vi "wait.vi"(8 "error_in":errorcluster, 11 "milliseconds_to_wait":u32) -> (0 "error_out":errorcluster)   [LabVIEW 2019]
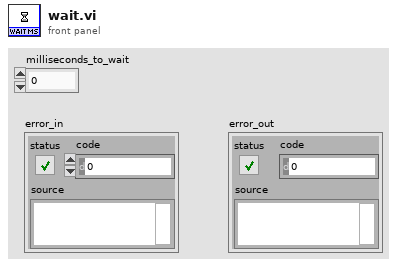
[diagram p1: front panel]
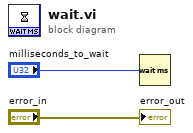
[diagram p0: block diagram]
diagram:
  n1 = Wait (ms)(milliseconds to wait="milliseconds_to_wait") -> ()  [unwired: 1 out]
  "error_out" <- "error_in"
